vi "Tensão.vi"() -> ()   [LabVIEW 2025]
panel:
  in  "Corrente":string
  in  "Toff":dbl
  in  "Ton(ms)":dbl
  out "Error out Fonte":errorcluster
  out "Error out Fonte":errorcluster
  in  "Passo_acrescimo(ms)":dbl
  in  "Tensão_Final":dbl
  in  "Acrescimo":dbl format="%#_6f"
  in  "Tensao_inicial":dbl format="%#_6p"
  in  "stop":bool
  in  "Endereço Agilent 6680A":i16
  out "Error out Fonte":errorcluster
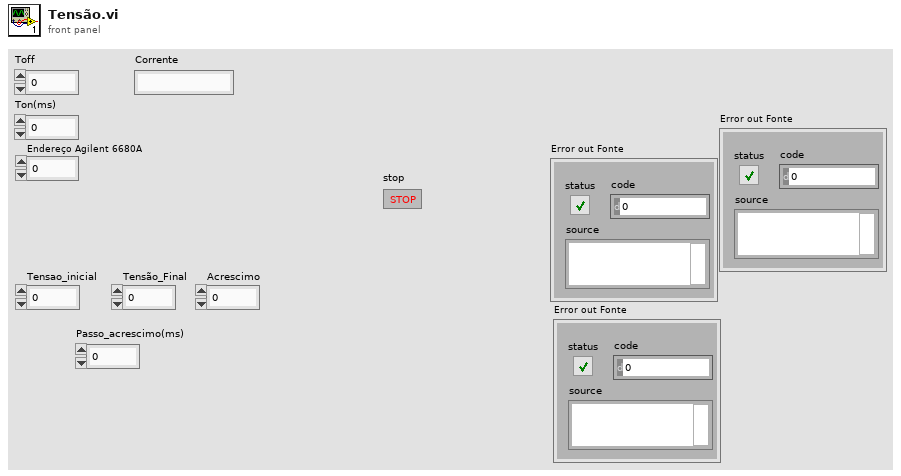
[diagram p1: front panel]
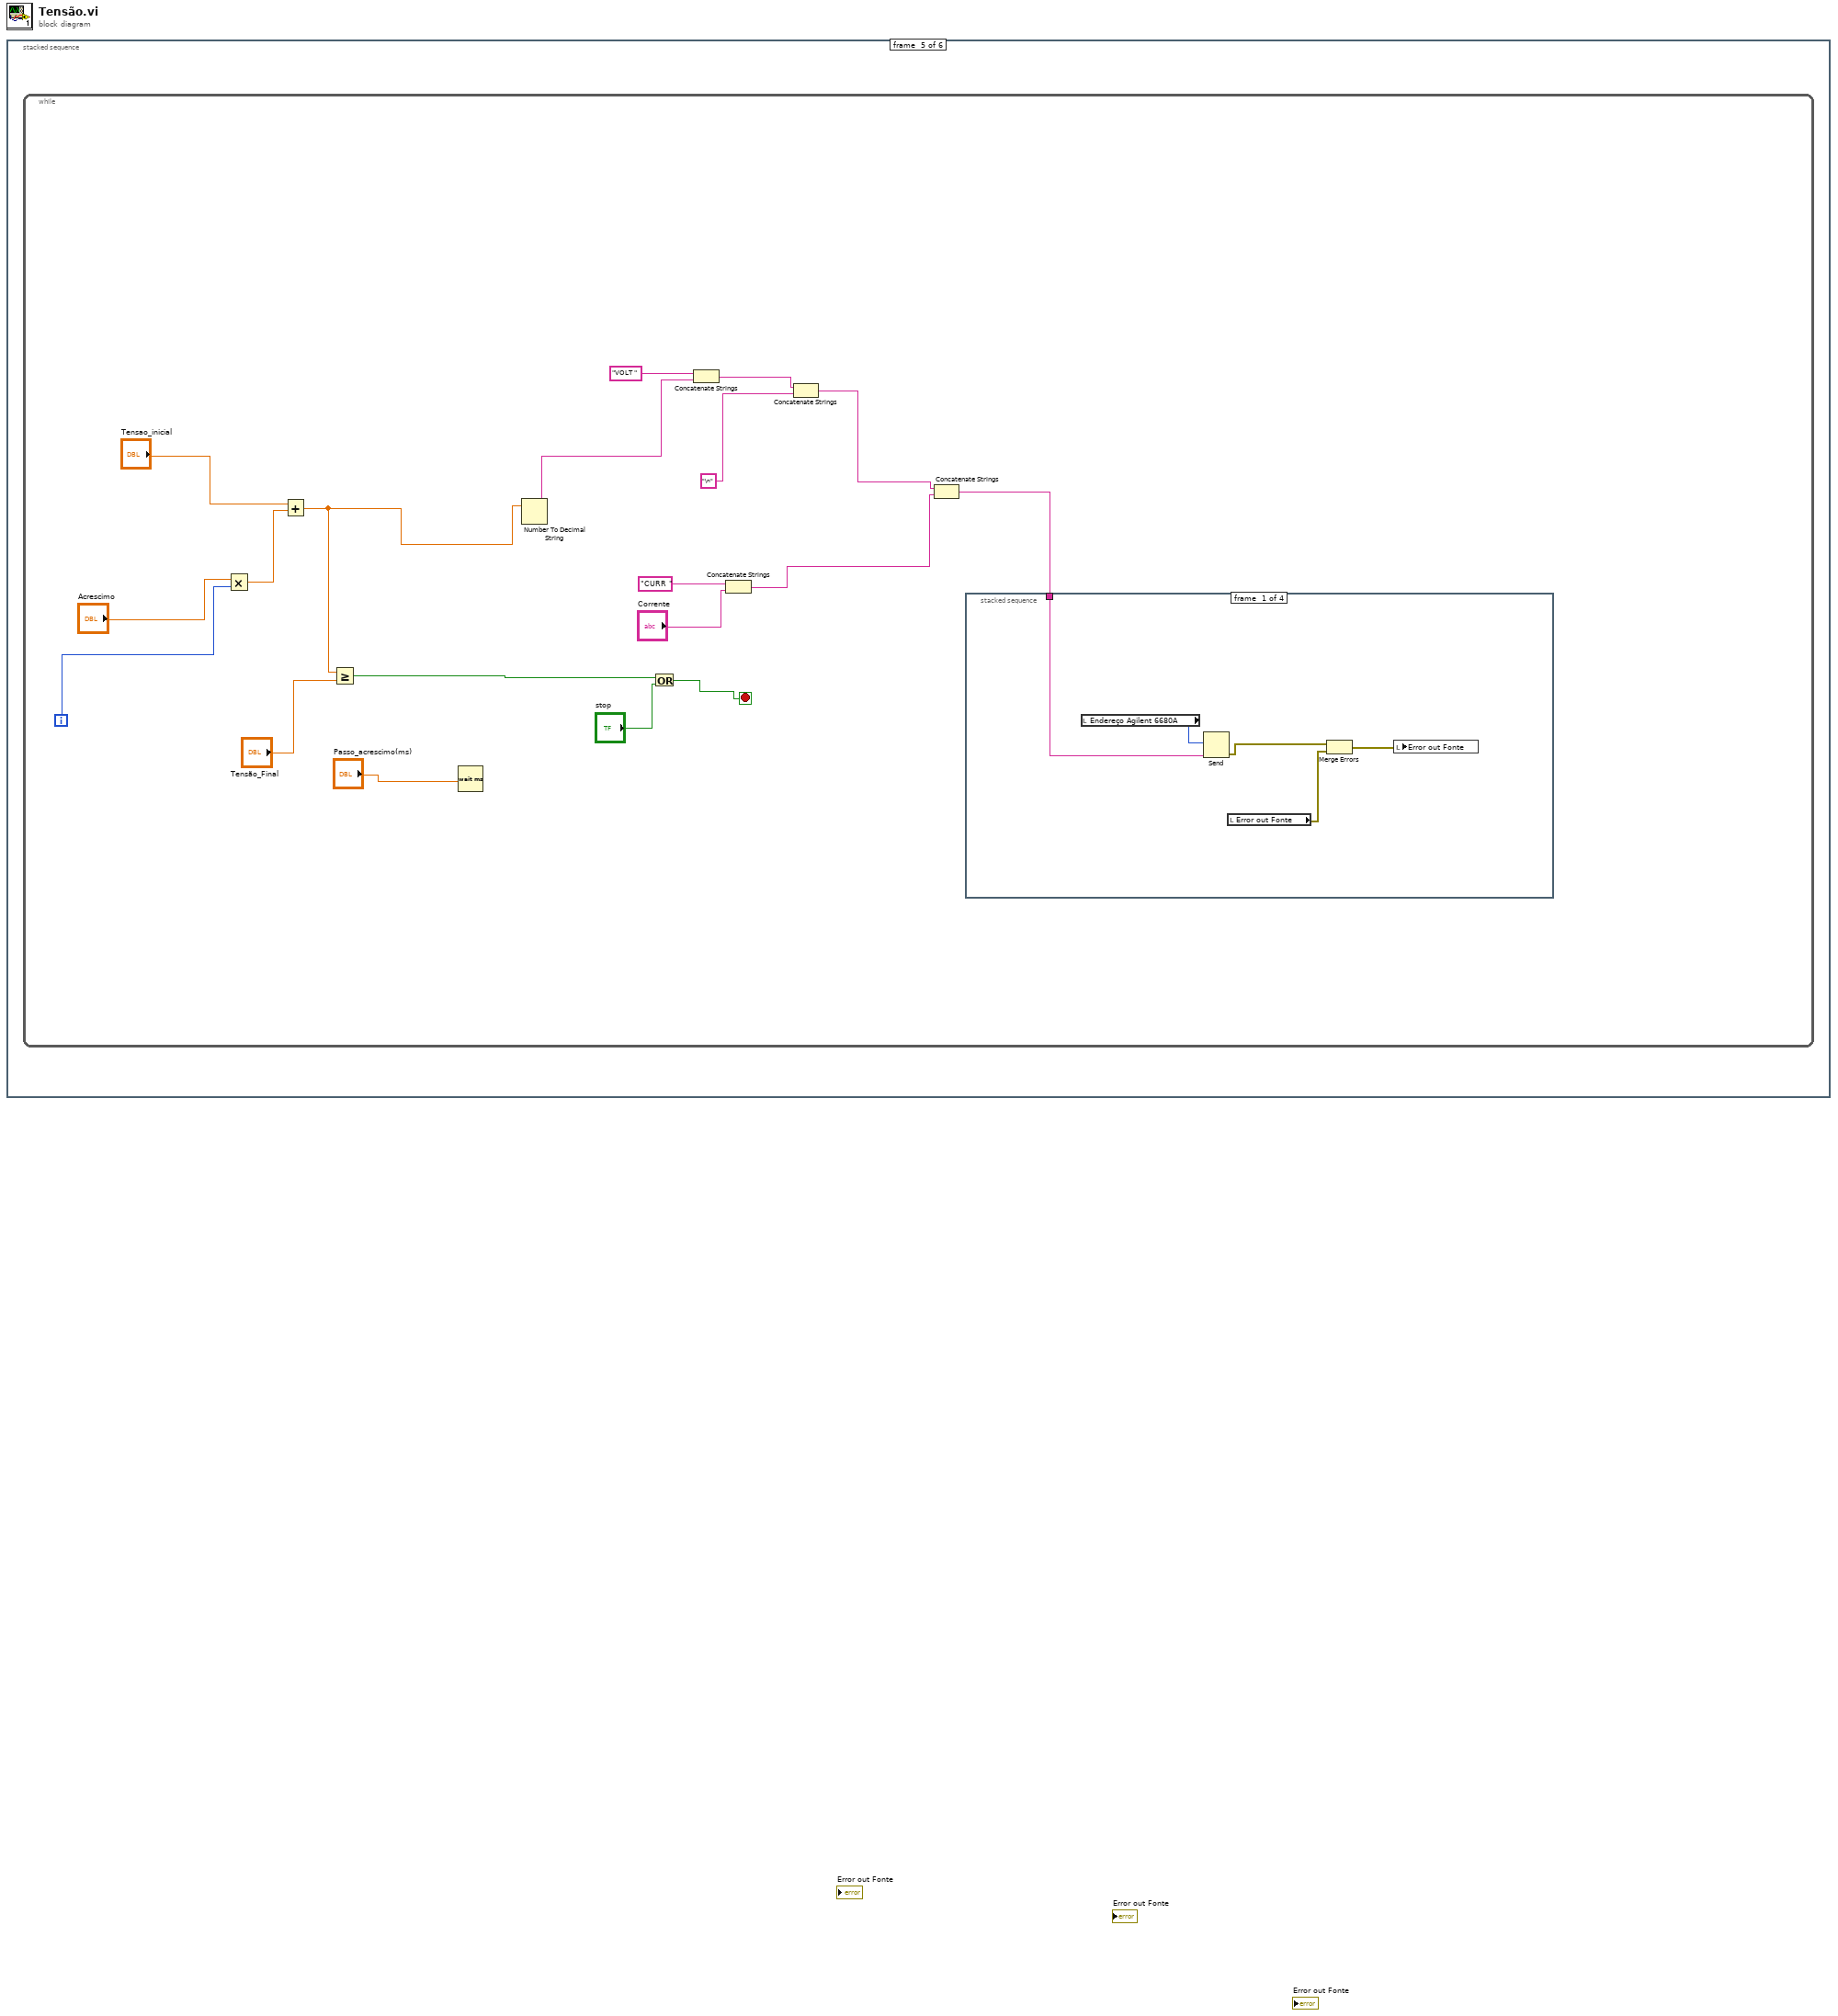
[diagram p0: block diagram]
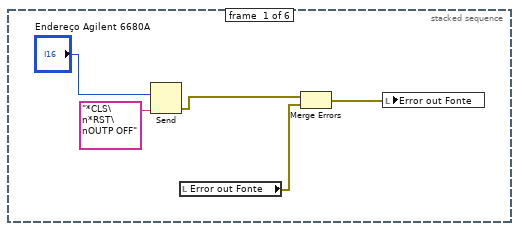
[diagram p2: hidden frame]
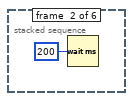
[diagram p3: hidden frame]
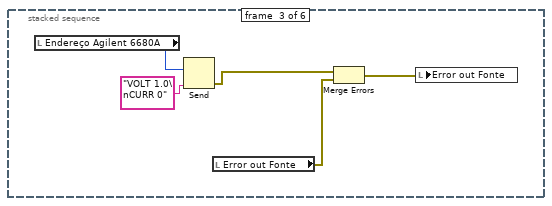
[diagram p4: hidden frame]
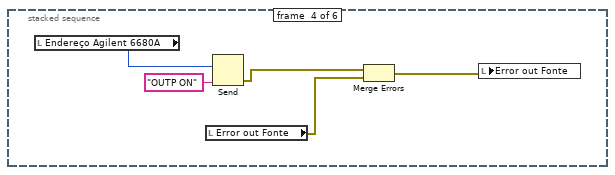
[diagram p5: hidden frame]
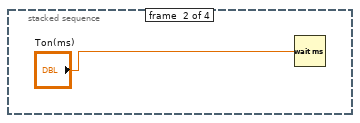
[diagram p6: hidden frame]
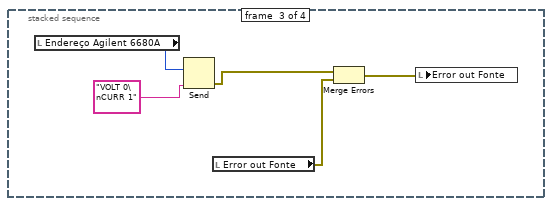
[diagram p7: hidden frame]
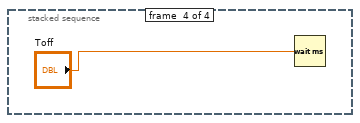
[diagram p8: hidden frame]
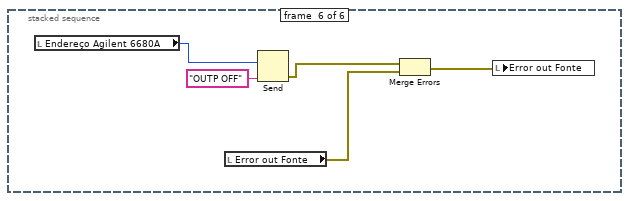
[diagram p9: hidden frame]
diagram:
  n1 = stacked-sequence {
    frame #0 {
      n2 = Send(2:"Endereço Agilent 6680A", 5:"*CLS\n*RST\nOUTP OFF" ("data string")) -> (8:w5:errorcluster)  [unwired: 3 in, 2 out]
      n3 = local read "Error out Fonte"() -> (w4:errorcluster)
      n4 = Merge Errors(w5, w4) -> (w1:errorcluster)
      n5 = local write "Error out Fonte"(w1) -> ()
    }
    frame #1 {
      n6 = Wait (ms)(milliseconds to wait=u32 200) -> ()  [unwired: 1 out]
    }
    frame #2 {
      n7 = local read "Endereço Agilent 6680A"() -> (w8:i16)
      n8 = Send(2:w8, 5:"VOLT 1.0\nCURR 0" ("data string")) -> (8:w10:errorcluster)  [unwired: 3 in, 2 out]
      n9 = local read "Error out Fonte"() -> (w11:errorcluster)
      n10 = Merge Errors(w10, w11) -> (w9:errorcluster)
      n11 = local write "Error out Fonte"(w9) -> ()
    }
    frame #3 {
      n12 = local read "Endereço Agilent 6680A"() -> (w12:i16)
      n13 = local read "Error out Fonte"() -> (w15:errorcluster)
      n14 = Send(2:w12, 5:"OUTP ON" ("data string")) -> (8:w14:errorcluster)  [unwired: 3 in, 2 out]
      n15 = Merge Errors(w14, w15) -> (w13:errorcluster)
      n16 = local write "Error out Fonte"(w13) -> ()
    }
    frame #4 {
      n17 = while {
        i -> [w27]
        stop <- w25 stop-if-true
        n18 = Multiply(x="Acrescimo", y=w27) -> (x*y=w32:dbl)
        n19 = Add(x="Tensao_inicial", y=w32) -> (x+y=w35:dbl)
        n20 = Greater Or Equal?(x=w35, y="Tensão_Final") -> (x >= y?=w34:bool)
        n21 = Wait (ms)(milliseconds to wait="Passo_acrescimo(ms)") -> ()  [unwired: 1 out]
        n22 = Number To Decimal String(number=w35) -> (decimal integer string=w17:string)  [unwired: 1 in]
        n23 = Or(x=w34, y="stop") -> (x .or. y?=w25:bool)
        n24 = Concatenate Strings("VOLT " ("data string"), w17) -> (w22:string)
        n25 = Concatenate Strings("CURR " ("data string"), "Corrente") -> (w20:string)
        n26 = Concatenate Strings(w22, "\n") -> (w21:string)
        n27 = Concatenate Strings(w21, w20) -> (w19:string)
        n28 = stacked-sequence {
          tunnel: w19 -> [w36 _ _ _]
          frame #0 {
            n29 = local read "Endereço Agilent 6680A"() -> (w40:i16)
            n30 = Send(2:w40, 5:w36) -> (8:w38:errorcluster)  [unwired: 3 in, 2 out]
            n31 = local read "Error out Fonte"() -> (w37:errorcluster)
            n32 = Merge Errors(w38, w37) -> (w39:errorcluster)
            n33 = local write "Error out Fonte"(w39) -> ()
          }
          frame #1 {
            n34 = Wait (ms)(milliseconds to wait="Ton(ms)") -> ()  [unwired: 1 out]
          }
          frame #2 {
            n35 = local read "Endereço Agilent 6680A"() -> (w46:i16)
            n36 = Send(2:w46, 5:"VOLT 0\nCURR 1" ("data string")) -> (8:w44:errorcluster)  [unwired: 3 in, 2 out]
            n37 = local read "Error out Fonte"() -> (w43:errorcluster)
            n38 = Merge Errors(w44, w43) -> (w45:errorcluster)
            n39 = local write "Error out Fonte"(w45) -> ()
          }
          frame #3 {
            n40 = Wait (ms)(milliseconds to wait="Toff") -> ()  [unwired: 1 out]
          }
        }
      }
    }
    frame #5 {
      n41 = local read "Endereço Agilent 6680A"() -> (w49:i16)
      n42 = local read "Error out Fonte"() -> (w50:errorcluster)
      n43 = Send(2:w49, 5:"OUTP OFF" ("data string")) -> (8:w51:errorcluster)  [unwired: 3 in, 2 out]
      n44 = Merge Errors(w51, w50) -> (w52:errorcluster)
      n45 = local write "Error out Fonte"(w52) -> ()
    }
  }
